vi "calcRequiredLoopTime_ticks.vi"(8 "error in (no error)":errorcluster, 11 "LoopTimer in":refnum<class "LoopTimer.lvclass">) -> (0 "error out":errorcluster, 3 "LoopTimer out":refnum<class "LoopTimer.lvclass">)   [LabVIEW 2013, in "ComponentData.lvlib" / "LoopTimer.lvclass"]
uses:
  <userlib>/Common/Component/Application/RT/ComponentData/LoopTimer/LoopTimer.lvclass
  <userlib>/Common/Component/Application/RT/ComponentData/LoopTimer/LoopTimer.lvclass/LoopTimer.ctl
  <userlib>/Common/Component/Application/RT/ComponentData/ConfigurationHandler/LoopConfig/LoopConfig.lvclass
  <userlib>/Common/Component/Application/RT/ComponentData/ConfigurationHandler/LoopInternalConfig/LoopInternalConfig.lvclass
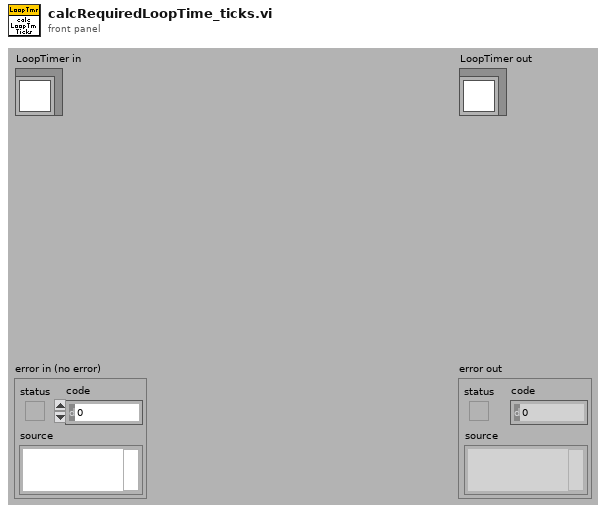
[diagram p1: front panel]
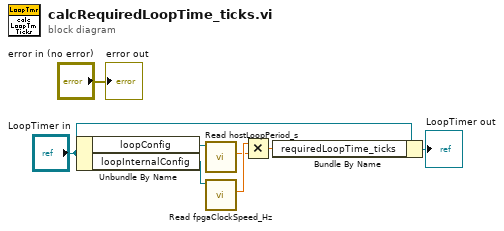
[diagram p0: block diagram]
diagram:
  n1 = Unbundle By Name("LoopTimer in") -> ("loopConfig"=w5:refnum<class "LoopConfig.lvclass">, "loopInternalConfig"=w4:refnum<class "LoopInternalConfig.lvclass">)
  n2 = call <userlib>:"Read hostLoopPeriod_s.vi"("LoopConfig in"=w5) -> ("hostLoopPeriod_s"=w2:dbl)  [unwired: 8 in, 2 out]
  n3 = call <userlib>:"Read fpgaClockSpeed_Hz.vi"("LoopConfigInternal in"=w4) -> ("fpgaClockSpeed_Hz"=w3:dbl)  [unwired: 8 in, 2 out]
  n4 = Multiply(x=w3, y=w2) -> (x*y=w1:dbl)
  n5 = Bundle By Name(cluster="LoopTimer in", "requiredLoopTime_ticks"=w1) -> (→"LoopTimer out":refnum<class "LoopTimer.lvclass">)
  "error out" <- "error in (no error)"
